vi "CLFNFixup.vi"   [LabVIEW 2020]
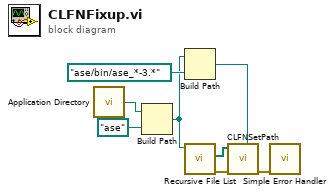
[diagram p0: block diagram]
diagram:
  n1 = call <vilib>:"Application Directory.vi"() -> ("Application Directory"=w3:path)
  n2 = Build Path(base path=w3, name or relative path=path "ase" ("base path")) -> (appended path=w2:path)
  n3 = Build Path(base path=w2, name or relative path=path "ase/bin/ase_*-3.*" ("New Path")) -> (appended path=w4:path)
  n4 = call <vilib>:"Recursive File List.vi"("Folder Path"=w2) -> ("error out"=w6:errorcluster, "All Files in Dir"=w8:path[])  [unwired: 6 in, 3 out]
  n5 = call "CLFNSetPath.vi"("New Path"=w4, "error in (no error)"=w6, "Files"=w8) -> ("error out"=w7:errorcluster)  [unwired: 7 in, 1 out]
  n6 = call <vilib>:"Simple Error Handler.vi"("error in (no error)"=w7) -> ()  [unwired: 4 in, 5 out]
